vi "ex_populateTreeFromDAQmxClasses.vi"(4 "error in (no error)":errorcluster, 5 "DAQmx classes":T8[](array[typedef]) {"Events"."Event Code" max=1073741823 step=1 format="%x"; "Methods"."Method Code" format="%x"; "Attributes"."Number of Dimensions" format="%x"; "Attributes"."Property Code" format="%x"}, 7 "tree ref":refnum<vi>) -> (0 "error out":errorcluster, 1 "DAQmx Channel Attributes":T1[](array[typedef]) {"Number of Dimensions" format="%x"; "Property Code" format="%x"}, 2 "DAQmx Channel Tags":string[](array[string]), 3 "dup tree ref":refnum<vi>)   [LabVIEW 2020]
uses:
  <vilib>/Platform/express/ex_EditUserDefinedProperties/controls.llb/ex_class3.ctl
  <vilib>/Platform/express/ex_EditUserDefinedProperties/controls.llb/ex_generictype3.ctl
  <vilib>/Platform/express/ex_EditUserDefinedProperties/controls.llb/ex_refnumenum.ctl
  <vilib>/Platform/express/ex_EditUserDefinedProperties/controls.llb/ex_cleanupenum.ctl
  <vilib>/Platform/express/ex_EditUserDefinedProperties/controls.llb/ex_yesnodefaultenum.ctl
  <vilib>/Platform/express/ex_EditUserDefinedProperties/controls.llb/ex_errorpassingenum.ctl
  <vilib>/Platform/express/ex_EditUserDefinedProperties/controls.llb/ex_matchexactenum.ctl
  <vilib>/Platform/express/ex_EditUserDefinedProperties/controls.llb/ex_callingenum.ctl
  <vilib>/Platform/express/ex_EditUserDefinedProperties/controls.llb/ex_filtering.ctl
  <vilib>/Platform/express/ex_EditUserDefinedProperties/controls.llb/ex_dialogenum.ctl
  <vilib>/Platform/express/ex_EditUserDefinedProperties/controls.llb/ex_attribute3.ctl
  <vilib>/Platform/express/ex_EditUserDefinedProperties/controls.llb/ex_datatypeenum.ctl
  <vilib>/Platform/express/ex_EditUserDefinedProperties/controls.llb/ex_clustercontrol.ctl
  <vilib>/Platform/express/ex_EditUserDefinedProperties/controls.llb/ex_enumeration.ctl
  <vilib>/Platform/express/ex_EditUserDefinedProperties/controls.llb/ex_yesnoenum.ctl
  <vilib>/Platform/express/ex_EditUserDefinedProperties/controls.llb/ex_accessenum.ctl
  <vilib>/Platform/express/ex_EditUserDefinedProperties/controls.llb/ex_initnameformat.ctl
  <vilib>/Platform/express/ex_EditUserDefinedProperties/controls.llb/ex_method3.ctl
  <vilib>/Platform/express/ex_EditUserDefinedProperties/controls.llb/ex_methflagsenum.ctl
  <vilib>/Platform/express/ex_EditUserDefinedProperties/controls.llb/ex_parameter2.ctl
  <vilib>/Platform/express/ex_EditUserDefinedProperties/controls.llb/ex_datanameenum.ctl
  <vilib>/Platform/express/ex_EditUserDefinedProperties/controls.llb/ex_numericdatatypeenum.ctl
  <vilib>/Platform/express/ex_EditUserDefinedProperties/controls.llb/ex_stringdatatypeenum.ctl
  <vilib>/Platform/express/ex_EditUserDefinedProperties/controls.llb/ex_passbyenum.ctl
  <vilib>/Platform/express/ex_EditUserDefinedProperties/controls.llb/ex_arrayfmtenum.ctl
  <vilib>/Platform/express/ex_EditUserDefinedProperties/controls.llb/ex_paraminoutenum.ctl
  <vilib>/Platform/express/ex_EditUserDefinedProperties/controls.llb/ex_eventdef.ctl
  <vilib>/Platform/express/ex_EditUserDefinedProperties/controls.llb/ex_eventparam.ctl
  <vilib>/Platform/express/ex_EditUserDefinedProperties/controls.llb/ex_eventparamtype.ctl
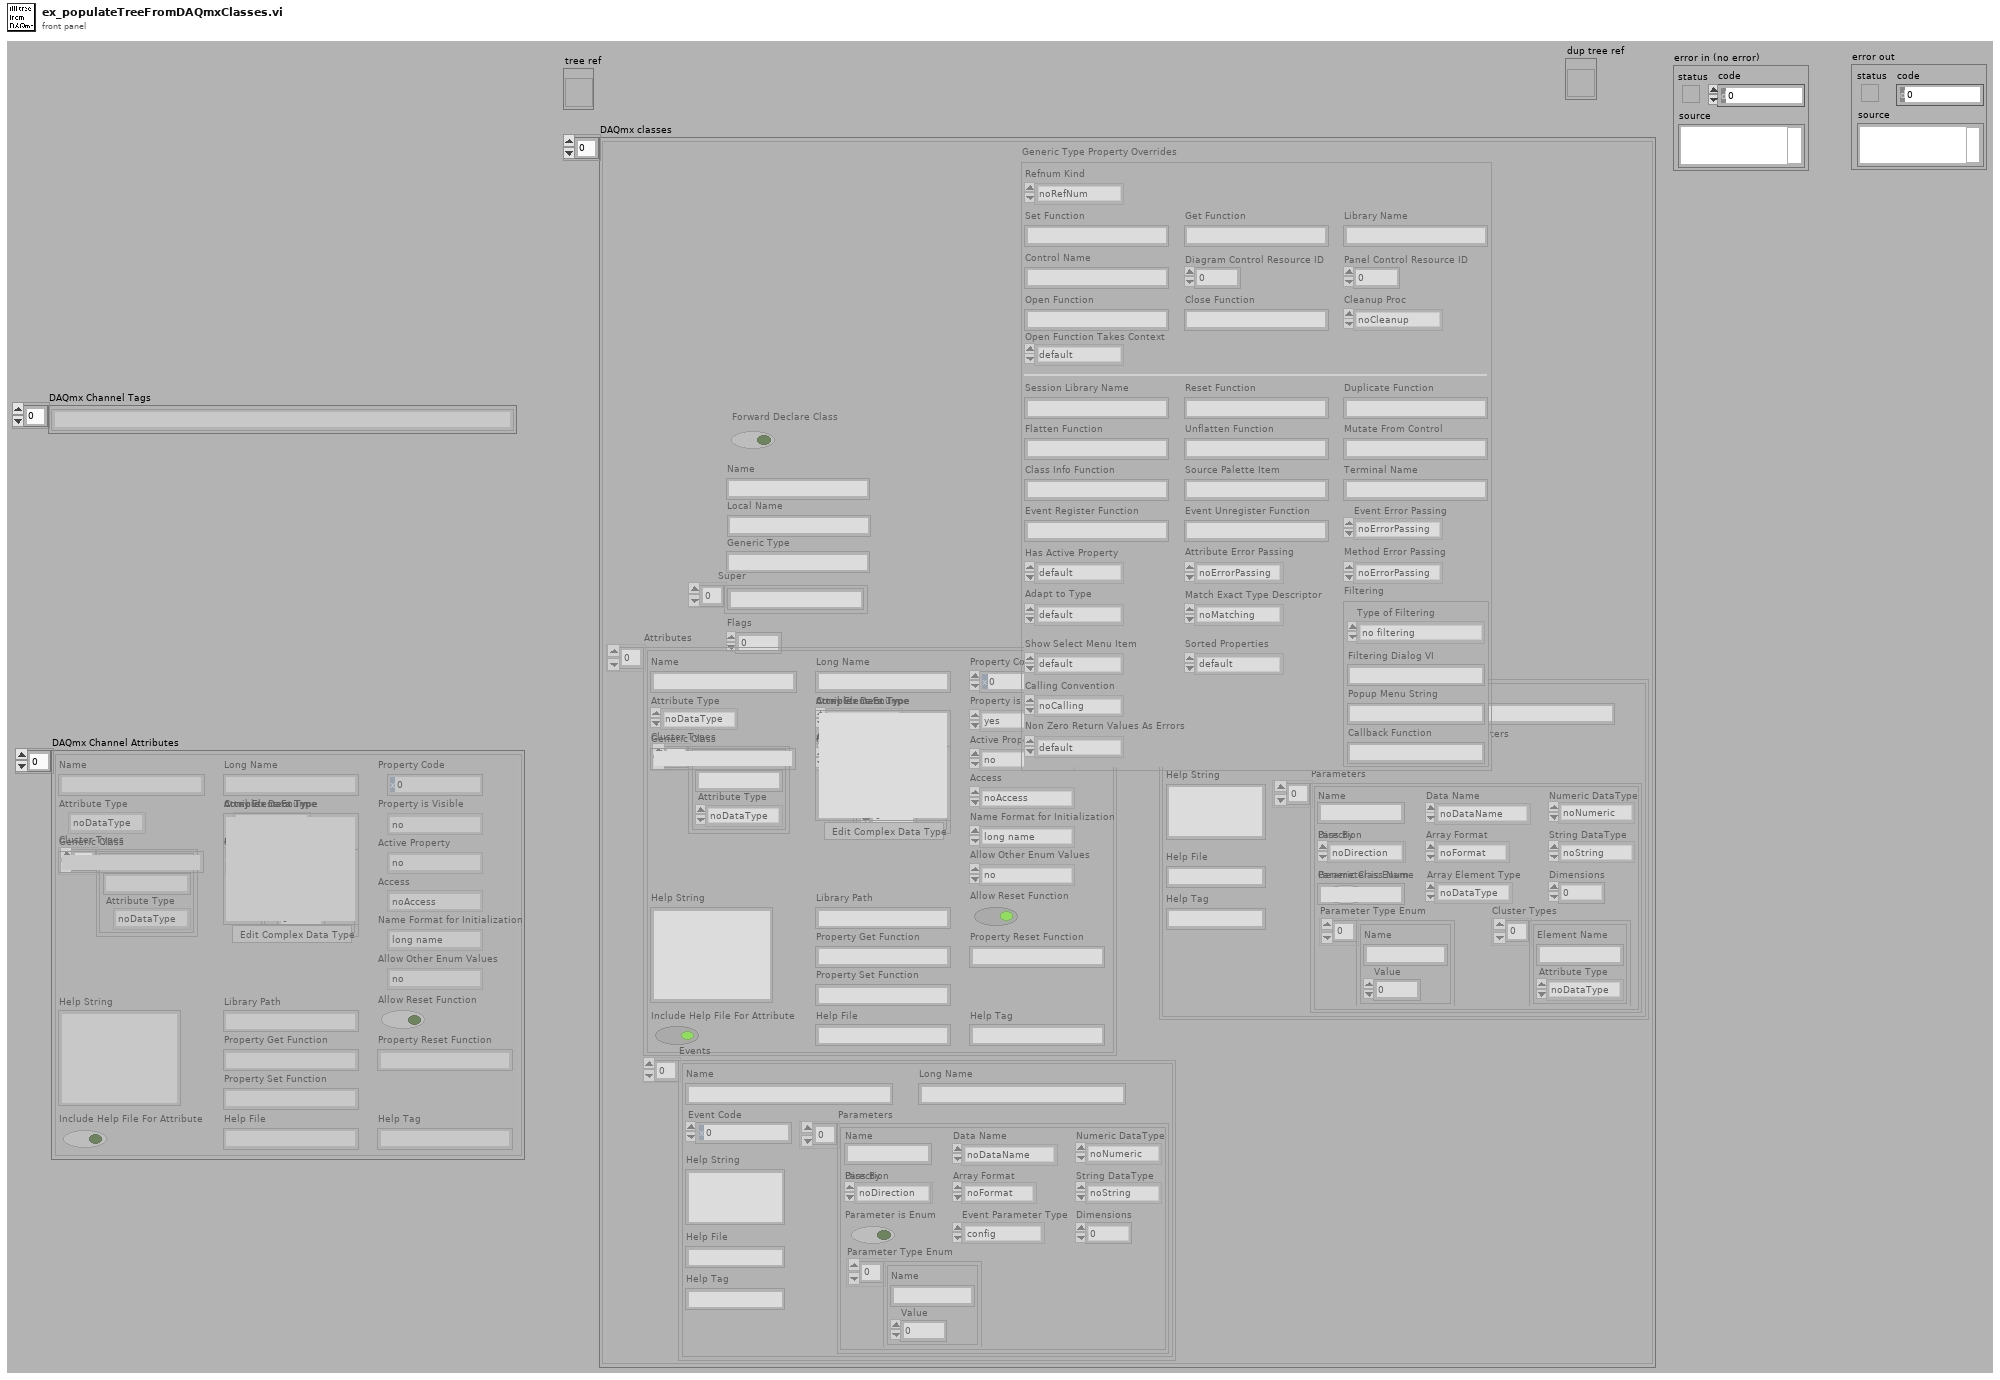
[diagram p1: front panel]
types:
  T1 = typedef "ex_attribute3.ctl" = cluster{"Name":string, "Long Name":string, "Property Code":i32, "Attribute Type":T2, "Cluster Types":T3[], "Attribute is Enum":bool, "Attribute Type Enum":T4[], "Property is Visible":T5, "Active Property":T5, "Access":T6, "Help String":string, "Library Path":string, "Property Get Function":string, "Property Set Function":string, "Allow Reset Function":bool, "Property Reset Function":string, "Generic Class":string, "Allow Other Enum Values":T5, "Array Element Type":T2, "Number of Dimensions":i32, "Complex Data Type":string, "Edit Complex Data Type":bool, "Name Format for Initialization":T7, "Include Help File For Attribute":bool, "Help Tag":string, "Help File":string}
  T2 = typedef "ex_datatypeenum.ctl" = enum16{"noDataType", "void", "iB", "iW", "iL", "iQ", "uB", "uW", "uL", "uQ", "fS", "fS1D", "fD", "fD1D", "bool", "bool1D", "string", "string1D", "path", "rect", "point", "VIRef", "VIRefReservation", "file", "VIExecState", "htmlImgFmt", "printFmt", "iW1D", "uW1D", "iL1D", "uL1D", "iQ1D", "uQ1D", "uB1D", "iB1D", "VisaRef", "DAQChannel", "DAQDevice", "DAQPhysChan", "DAQScale", "DAQSwitch", "DAQTask", "DAQTerminal", "DAQTrigger", "cluster", "genclass", "timestamp", "array", "variant", "complex type"}
  T3 = typedef "ex_clustercontrol.ctl" = cluster{"Element Name":string, "Attribute Type":T2}
  T4 = typedef "ex_enumeration.ctl" = cluster{"Name":string, "Value":i32}
  T5 = typedef "ex_yesnoenum.ctl" = enum16{"no", "yes"}
  T6 = typedef "ex_accessenum.ctl" = enum16{"noAccess", "readwrite", "readonly", "writeonly"}
  T7 = typedef "ex_initnameformat.ctl" = enum16{"long name", "short name"}
  T8 = typedef "ex_class3.ctl" = cluster{"Name":string, "Local Name":string, "Generic Type":string, "Super":string[], "Forward Declare Class":bool, "Flags":i32, "Generic Type Property Overrides":T9, "Attributes":T1[], "Methods":T18[], "Events":T27[]}
  T9 = typedef "ex_generictype3.ctl" = cluster{"Refnum Kind":T10, "Set Function":string, "Get Function":string, "Library Name":string, "Control Name":string, "Diagram Control Resource ID":i32, "Panel Control Resource ID":i32, "Open Function":string, "Close Function":string, "Cleanup Proc":T11, "Open Function Takes Context":T12, "Session Library Name":string, "Reset Function":string, "Duplicate Function":string, "Flatten Function":string, "Unflatten Function":string, "Mutate From Control":string, "Class Info Function":string, "Source Palette Item":string, "Terminal Name":string, "Event Register Function":string, "Event Unregister Function":string, "Event Error Passing":T13, "Has Active Property":T12, "Attribute Error Passing":T13, "Method Error Passing":T13, "Adapt to Type":T12, "Match Exact Type Descriptor":T14, "Show Select Menu Item":T12, "Sorted Properties":T12, "Calling Convention":T15, "Filtering":T16, "Non Zero Return Values As Errors":T12}
  T10 = typedef "ex_refnumenum.ctl" = enum16{"noRefNum", "Generic", "GenericTag", "GenericByValue", "GenericByRefFlatten", "GenericTagByRefFlatten"}
  T11 = typedef "ex_cleanupenum.ctl" = enum16{"noCleanup", "exit", "idle", "reset", "idleNotTop", "resetNotTop", "doNotCleanup"}
  T12 = typedef "ex_yesnodefaultenum.ctl" = enum16{"default", "no", "yes"}
  T13 = typedef "ex_errorpassingenum.ctl" = enum16{"noErrorPassing", "none", "stringFirst", "stringLast"}
  T14 = typedef "ex_matchexactenum.ctl" = enum16{"noMatching", "none", "withInheritance", "strict"}
  T15 = typedef "ex_callingenum.ctl" = enum16{"noCalling", "std", "C"}
  T16 = typedef "ex_filtering.ctl" = cluster{"Type of Filtering":T17, "Filtering Dialog VI":string, "Popup Menu String":string, "Callback Function":string}
  T17 = typedef "ex_dialogenum.ctl" = enum16{"no filtering", "filtering", "ipfiltering"}
  T18 = typedef "ex_method3.ctl" = cluster{"Name":string, "Local Name":string, "Method Flags":T19, "Method Code":i32, "# Optional Parameters":i32, "Parameters":T20[], "Help String":string, "Help Tag":string, "Help File":string}
  T19 = typedef "ex_methflagsenum.ctl" = enum16{"noFlags", "noInvoke", "returnValue", "returnErrClustCode", "0", "retErrClustNoInv"}
  T20 = typedef "ex_parameter2.ctl" = cluster{"Name":string, "Data Name":T21, "Numeric DataType":T22, "String DataType":T23, "Dimensions":u32, "Pass By":T24, "Array Format":T25, "Parameter is Enum":bool, "Parameter Type Enum":T4[], "Cluster Types":T3[], "Generic Class Name":string, "Array Element Type":T2, "Direction":T26}
  T21 = typedef "ex_datanameenum.ctl" = enum16{"noDataName", "numeric", "array", "string", "void", "error", "cluster", "genclass", "timestamp", "variant", "non numeric array", "bool", "path"}
  T22 = typedef "ex_numericdatatypeenum.ctl" = enum16{"noNumeric", "int8", "int16", "int32", "int64", "uInt8", "uInt16", "uInt32", "uInt64", "single", "double"}
  T23 = typedef "ex_stringdatatypeenum.ctl" = enum16{"noString", "CStr", "PStr", "StrHandle", "StrHandlePtr"}
  T24 = typedef "ex_passbyenum.ctl" = enum16{"noPassing", "value", "reference", "refInOut"}
  T25 = typedef "ex_arrayfmtenum.ctl" = enum16{"noFormat", "pointer", "handle", "handlepointer"}
  T26 = typedef "ex_paraminoutenum.ctl" = enum16{"noDirection", "in", "out", "inout"}
  T27 = typedef "ex_eventdef.ctl" = cluster{"Name":string, "Long Name":string, "Event Code":u32, "Parameters":T28[], "Help String":string, "Help Tag":string, "Help File":string}
  T28 = typedef "ex_eventparam.ctl" = cluster{"Name":string, "Data Name":T21, "Numeric DataType":T22, "String DataType":T23, "Dimensions":u32, "Pass By":T24, "Array Format":T25, "Parameter is Enum":bool, "Parameter Type Enum":T4[], "Direction":T26, "Event Parameter Type":T29}
  T29 = typedef "ex_eventparamtype.ctl" = enum16{"config", "data", "configdata"}
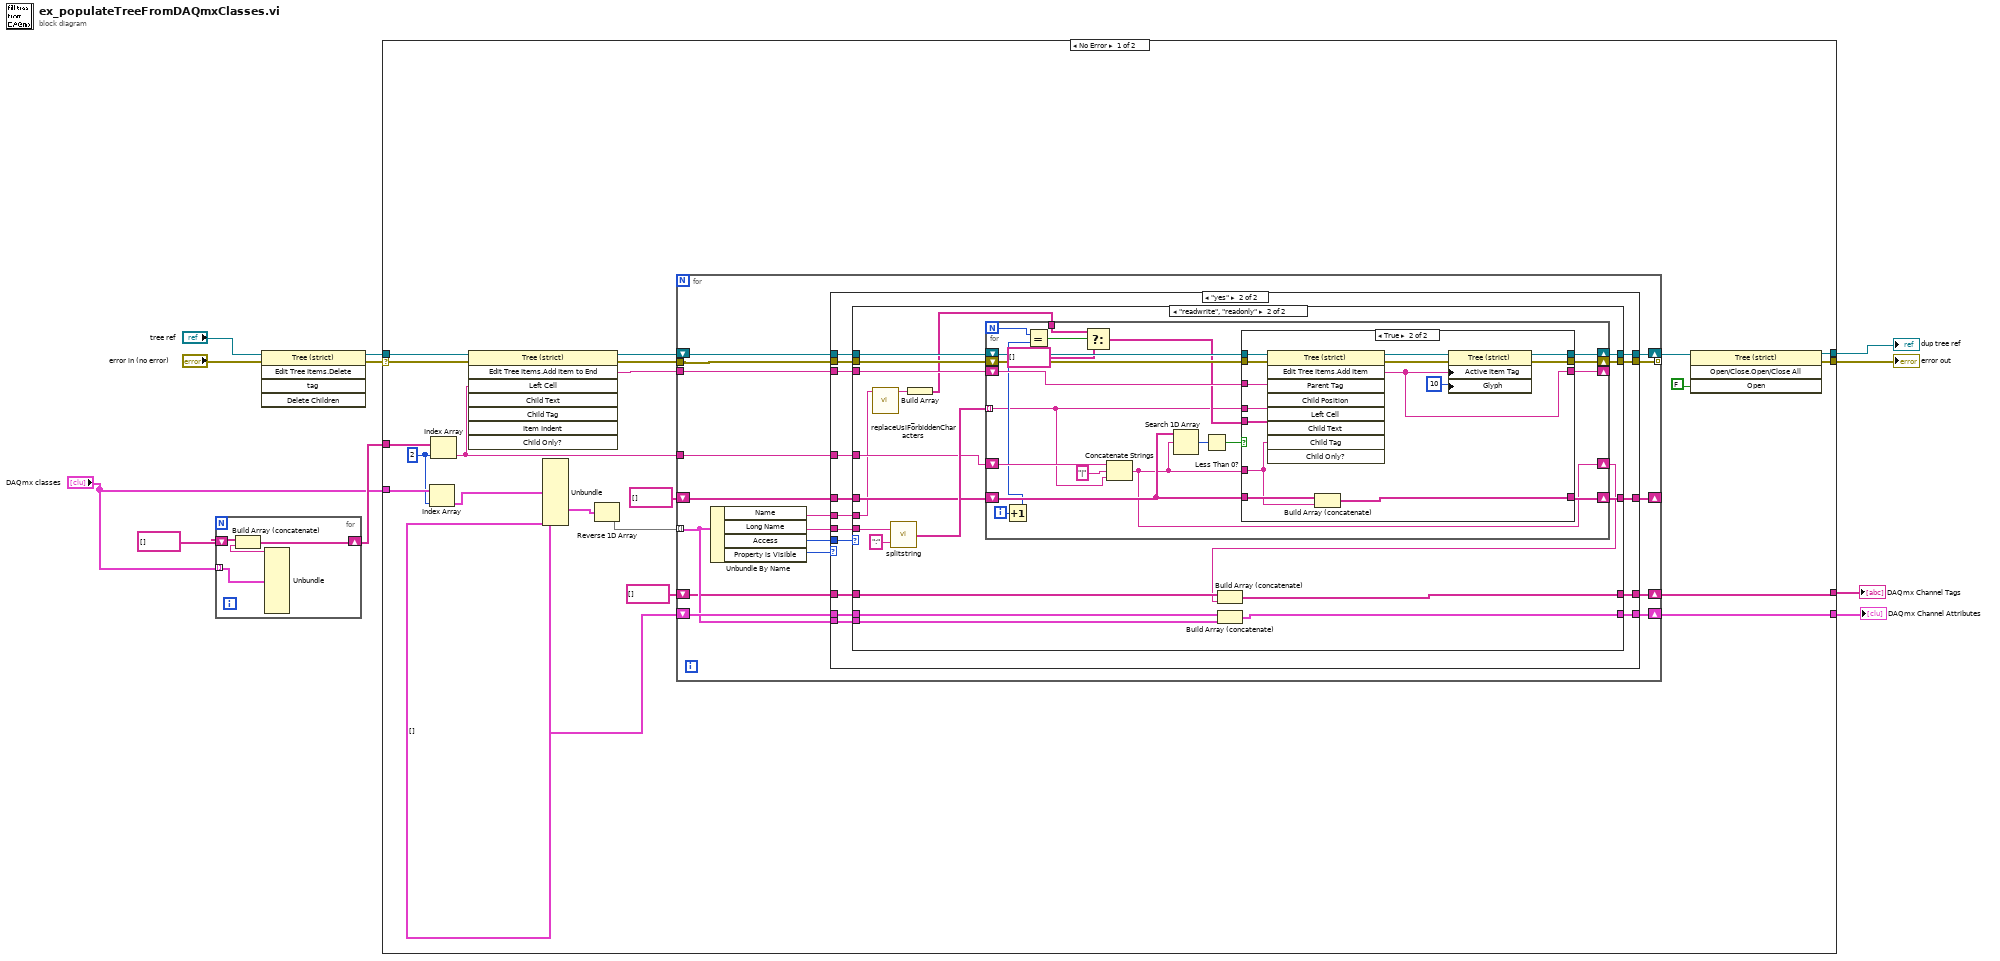
[diagram p0: block diagram]
diagram:
  n1 = for {
    tunnel: "DAQmx classes" -> [w13] mode=indexing
    shift-right: [w15] -> w2
    shift-left: string[] [] -> [w14]
    n2 = Unbundle(w13) -> ("Name"=w12:string)  [unwired: 9 out]
    n3 = Build Array (concatenate)(w14, w12) -> (w15:string[])
  }
  n4 = invoke class="Tree (strict)" method="Edit Tree Items.Delete"(reference="tree ref", error in="error in (no error)") -> (reference out=w9:refnum<vi>, error out=w11:errorcluster)  [unwired: 3 in, 3 out]
  n5 = case shown="No Error" w11 {
    selector: w11 -> [w22 w139]
    tunnel: w9 -> [w36 w140]
    tunnel: [w26 w139] -> w6
    tunnel: w2 -> [w27 _]
    tunnel: "DAQmx classes" -> [w25 _]
    tunnel: [w21 w140] -> w8
    tunnel: [w19 _] -> w5
    tunnel: [w18 _] -> w4
    frame No Error {
      w23 = 2 ("index (row)")
      n6 = Index Array(array=w25, index=w23) -> (element=w24:T8)
      n7 = Index Array(array=w27, index=w23) -> (element=w28:string)
      n8 = invoke on="Invoke Node" class="Tree (strict)" method="Edit Tree Items.Add Item to End"(reference=w36, error in=w22, "Left Cell"=w28) -> (reference out=w33:refnum<vi>, error out=w32:errorcluster, "Edit Tree Items:Add Item to End"=w17:string)  [unwired: 5 in, 5 out]
      n9 = Unbundle(w24) -> ("Attributes"=w20:T1[])  [unwired: 9 out]
      n10 = Reverse 1D Array(array=w20) -> (reversed array=w30:T1[])
      n11 = for {
        tunnel: w30 -> [w40] mode=indexing
        tunnel: w32 -> [w51]
        tunnel: [w50] -> _ mode=indexing
        tunnel: w17 -> [w49]
        shift-right: [w48] -> _
        shift-left: string[] [] -> [w47]
        shift-right: [w46] -> w35
        shift-left: w33 -> [w52]
        tunnel: w28 -> [w44]
        shift-right: [w41] -> w19
        shift-left: T1[] [] -> [w42]
        shift-right: [w37] -> w18
        shift-left: string[] [] -> [w38]
        n12 = Unbundle By Name(w40) -> ("Name"=w43:string, "Long Name"=w53:string, "Access"=w45:T6, "Property is Visible"=w39:T5)
        n13 = case shown="\"yes\"" w39 {
          tunnel: w53 -> [_ w74]
          tunnel: w52 -> [w55 w73]
          tunnel: w51 -> [w56 w72]
          tunnel: [w56 w71] -> w50
          tunnel: w49 -> [_ w70]
          tunnel: [w57 w69] -> w48
          tunnel: w47 -> [w57 w68]
          tunnel: [w55 w67] -> w46
          tunnel: w45 -> [_ w66]
          tunnel: w44 -> [_ w65]
          tunnel: w43 -> [_ w64]
          tunnel: w42 -> [w58 w63]
          tunnel: [w58 w62] -> w41
          tunnel: w40 -> [_ w61]
          tunnel: w38 -> [w54 w60]
          tunnel: [w54 w59] -> w37
          frame "no", Default {
          }
          frame "yes" {
            n14 = case shown="\"readwrite\", \"readonly\"" w66 {
              tunnel: w74 -> [_ w89]
              tunnel: w73 -> [w79 w99]
              tunnel: w72 -> [w78 w98]
              tunnel: [w78 w97] -> w71
              tunnel: w70 -> [_ w95]
              tunnel: [w77 w94] -> w69
              tunnel: w68 -> [w77 w93]
              tunnel: [w79 w92] -> w67
              tunnel: w65 -> [_ w91]
              tunnel: w64 -> [_ w84]
              tunnel: w63 -> [w76 w88]
              tunnel: [w76 w87] -> w62
              tunnel: w61 -> [_ w86]
              tunnel: w60 -> [w75 w82]
              tunnel: [w75 w81] -> w59
              frame Default {
              }
              frame "readwrite", "readonly" {
                n15 = call <vilib>:"_replaceUsiForbiddenCharacters.vi"("string in"=w84) -> ("string out"=w83:string)  [unwired: 5 in, 1 out]
                n16 = call <vilib>:"splitstring.vi"("search string/char (-)"=":", "string"=w89) -> ("Array"=w96:string[])
                n17 = Build Array(w83) -> (w90:string[])
                n18 = for {
                  N -> [w106]
                  tunnel: w96 -> [w100] mode=indexing
                  shift-right: [w116] -> _
                  shift-left: w95 -> [w117]
                  shift-right: [w111] -> w80
                  shift-left: w91 -> [w115]
                  shift-right: [w113] -> w94
                  shift-left: w93 -> [w112]
                  shift-right: [w108] -> w92
                  shift-left: w99 -> [w120]
                  shift-right: [w118] -> w97
                  shift-left: w98 -> [w119]
                  tunnel: w90 -> [w103]
                  i -> [w107]
                  n19 = Increment(x=w107) -> (x+1=w105:i32)
                  n20 = Equal?(x=w106, y=w105) -> (x = y?=w104:bool)
                  n21 = Select(t=w103, s=w104, f=string[] []) -> (s? t:f=w101:string[])
                  n22 = Concatenate Strings(w115, "|" ("search string/char (-)"), w100) -> (w111:string)
                  n23 = Search 1D Array(1D array=w112, element=w111) -> (index of element=w110:i32)  [unwired: 1 in]
                  n24 = Less Than 0?(x=w110) -> (x < 0?=w109:bool)
                  n25 = case shown="True" w109 {
                    tunnel: w120 -> [w121 w138]
                    tunnel: w119 -> [w124 w137]
                    tunnel: [w124 w127] -> w118
                    tunnel: w117 -> [_ w136]
                    tunnel: [w122 w130] -> w116
                    tunnel: w100 -> [_ w135]
                    tunnel: w112 -> [w123 w134]
                    tunnel: w111 -> [w122 w133]
                    tunnel: [w123 w132] -> w113
                    tunnel: [w121 w125] -> w108
                    tunnel: w101 -> [_ w131]
                    frame False {
                    }
                    frame True {
                      n26 = invoke on="Invoke Node" class="Tree (strict)" method="Edit Tree Items.Add Item"(reference=w138, error in=w137, "Parent Tag"=w136, "Left Cell"=w135, "Child Text"=w131, "Child Tag"=w133) -> (reference out=w126:refnum<vi>, error out=w128:errorcluster, "Edit Tree Items:Add Item"=w130:string)  [unwired: 3 in, 6 out]
                      n27 = Build Array (concatenate)(w134, w133) -> (w132:string[])
                      n28 = property class="Tree (strict)"(reference=w126, error in=w128, "Active Item Tag"=w130, "Glyph"=10 ("Active Item:Symbol Index")) -> (reference out=w125:refnum<vi>, error out=w127:errorcluster)
                    }
                  }
                }
                n29 = Build Array (concatenate)(w82, w80) -> (w81:string[])
                n30 = Build Array (concatenate)(w88, w86) -> (w87:T1[])
              }
            }
          }
        }
      }
      n31 = invoke on="Invoke Node" class="Tree (strict)" method="Open/Close.Open/Close All"(reference=w35, "Open"=FALSE ("Open?")) -> (reference out=w21:refnum<vi>, error out=w26:errorcluster)  [unwired: 2 in, 2 out]
    }
    frame Error {
    }
  }
  "error out" <- w6
  "dup tree ref" <- w8
  "DAQmx Channel Attributes" <- w5
  "DAQmx Channel Tags" <- w4
